vi "IMIC_GetYPos.vi"(0 "handle":u64) -> (1 "output param":T1(ring), 2 "handle out":u64, 3 "xpos":dbl)   [LabVIEW 2011]
uses:
  tillimic64.dll
panel:
  # "never used"
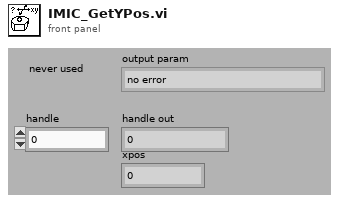
[diagram p1: front panel]
types:
  T1 = enum16{"no error", "missing axis", "missing Z axis", "missing Filter", "iMic not initialized", "no property", "wrong handle", "protocol not finished", "user parameter to long (>32 bits)", "no user parameter handle", "failed to open comport", "failed to initialize"}
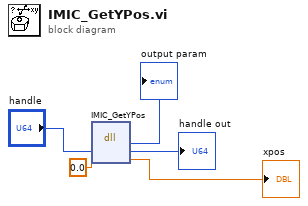
[diagram p0: block diagram]
diagram:
  n1 = dll-call lib="C:/Program Files/colibri/Drivers/TILLPhotonics/tillimic*.*" fn="IMIC_GetYPos"("handle"="handle", "xpos"=0.0 ("zpos")) -> ("return type"=→"output param":i32, "handle"=→"handle out":u64, "xpos"=→"xpos":dbl)  [unwired: 3 in, 2 out]
